vi "Configure Sequence.vi"   [LabVIEW 2016, in "Agilent N6700 Series.lvlib"]
doc: "Configures a current or voltage sequence.\n\n<b>Note:</b>\n\nThis VI only applies to the N6705B DC Power Analyzer."
uses:
  <instrlib>/Agilent N6700 Series/Agilent N6700 Series.lvlib
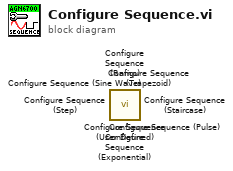
[diagram p0: block diagram]
diagram:
  n1 = call <instrlib>:"Configure Sequence (User Defined).vi"() -> ()  [unwired: 18 in, 2 out]
  n2 = call <instrlib>:"Configure Sequence (Trapezoid).vi"() -> ()  [unwired: 18 in, 2 out]
  n3 = call <instrlib>:"Configure Sequence (Step).vi"() -> ()  [unwired: 18 in, 2 out]
  n4 = call <instrlib>:"Configure Sequence (Staircase).vi"() -> ()  [unwired: 18 in, 2 out]
  n5 = call <instrlib>:"Configure Sequence (Sine Wave).vi"() -> ()  [unwired: 18 in, 2 out]
  n6 = call <instrlib>:"Configure Sequence (Ramp).vi"() -> ()  [unwired: 18 in, 2 out]
  n7 = call <instrlib>:"Configure Sequence (Pulse).vi"() -> ()  [unwired: 18 in, 2 out]
  n8 = call <instrlib>:"Configure Sequence (Exponential).vi"() -> ()  [unwired: 18 in, 2 out]
